vi "Write Startup Configuration.vi"(8 "error in (no error)":errorcluster, 10 "Initial Configuration":T1={"Load Modules"=[enum."Monitor Controller", enum."Pulse Controller", enum."VISA Device", enum."NI-DAQmx", enum."NI-Scope", enum."Red Pitaya Digitizer", enum."Red Pitaya Lockin", enum."Integrate Pulse", enum."Lockin Processor", enum."File converter", enum."NHMFL Synthesizer"]}, 11 "Application Controller in":refnum<class "Application Controller.lvclass">) -> (0 "error out":errorcluster, 3 "Application Controller out":refnum<class "Application Controller.lvclass">)   [LabVIEW 2016, in "Application Controller.lvclass"]
uses:
  Application Controller.lvclass
  Measure_extentions/Monitor-Pulse/Start-up Configuration.ctl
  Measure_extentions/Monitor-Pulse/Module Types.ctl
  Application Controller.lvclass/Application Controller.ctl
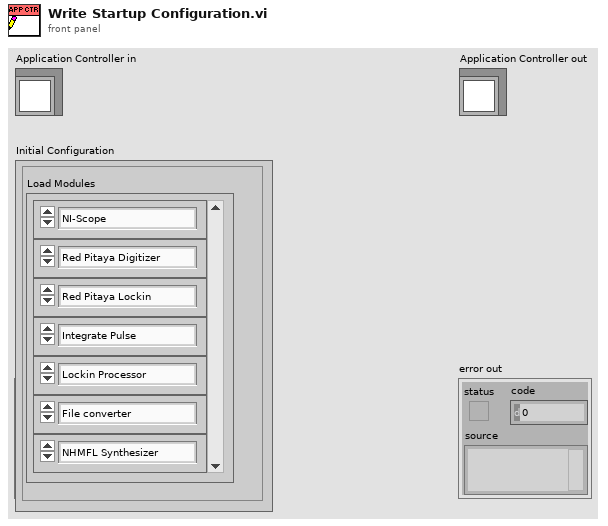
[diagram p1: front panel]
types:
  T1 = typedef "Start-up Configuration.ctl" = cluster{"Load Modules":T2[]}
  T2 = typedef "Module Types.ctl" = enum16{"NONE", "NI-DAQmx", "NI-Scope", "Red Pitaya Digitizer", "GaGe", "VISA Device", "Red Pitaya Lockin", "Monitor Controller", "Pulse Controller", "Integrate Pulse", "Lockin Processor", "File converter", "NHMFL Synthesizer", "Micron Hyperion", "Spectrum Recorder"}
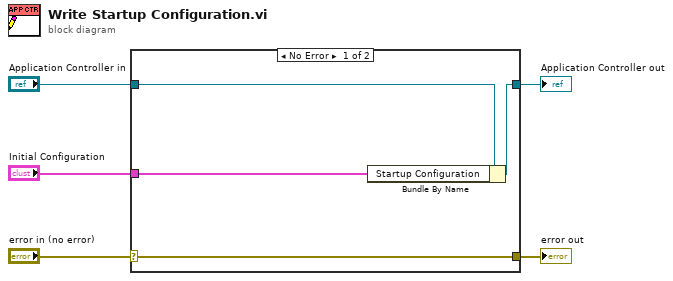
[diagram p0: block diagram]
diagram:
  n1 = case shown="No Error" "error in (no error)" {
    selector: "error in (no error)" -> [w9 w10]
    tunnel: [w9 w10] -> w4
    tunnel: [w7 w11] -> w2
    tunnel: "Application Controller in" -> [w8 w11]
    tunnel: "Initial Configuration" -> [w6 _]
    frame No Error {
      n2 = Bundle By Name(cluster=w8, "Startup Configuration"=w6) -> (w7:refnum<class "Application Controller.lvclass">)
    }
    frame Error {
    }
  }
  "error out" <- w4
  "Application Controller out" <- w2
